vi "Coerce Scale Range to Content.vi"(8 "error in (no error)":errorcluster, 11 "Base Graph in":refnum<class "Base Graph.lvclass">) -> (0 "error out":errorcluster, 3 "Base Graph out":refnum<class "Base Graph.lvclass">)   [LabVIEW 2023, in "Base Graph.lvclass"]
uses:
  Base Graph.lvclass
  Base Graph.lvclass/Base Graph.ctl
panel:
  # "AFTER DEZOOMING THE INTENSITY GRAPH IS 1PIXEL TO BIG"
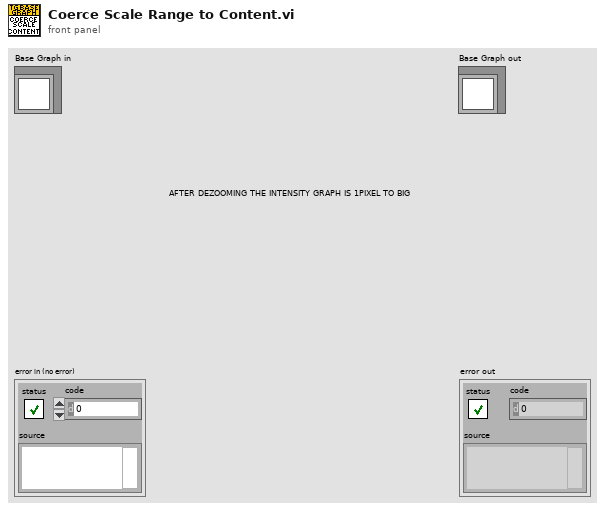
[diagram p1: front panel]
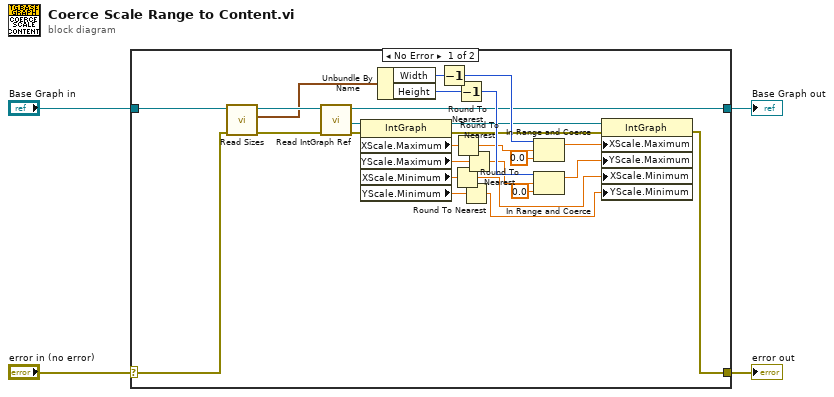
[diagram p0: block diagram]
diagram:
  n1 = case shown="No Error" "error in (no error)" {
    selector: "error in (no error)" -> [w26 w33]
    tunnel: [w13 w33] -> w3
    tunnel: [w14 w32] -> w1
    tunnel: "Base Graph in" -> [w31 w32]
    frame No Error {
      n2 = call "Read Sizes.vi"("error in (no error)"=w26, "TG Base Graph in"=w31) -> ("error out"=w27:errorcluster, "Sizes"=w28:cluster{"Height":u32, "Width":u32}, "TG Base Graph out"=w30:refnum<class "Base Graph.lvclass">)  [unwired: 7 in]
      n3 = call "Read IntGraph Ref.vi"("error in (no error)"=w27, "TG Base Graph in"=w30) -> ("error out"=w25:errorcluster, "IntGraph Ref"=w29:refnum<vi>, "TG Base Graph out"=w14:refnum<class "Base Graph.lvclass">)  [unwired: 7 in]
      n4 = property class="IntGraph"(reference=w29, error in=w25) -> (reference out=w16:refnum<vi>, error out=w15:errorcluster, "XScale.Maximum"=w24:dbl, "YScale.Maximum"=w20:dbl, "XScale.Minimum"=w10:dbl, "YScale.Minimum"=w9:dbl)
      n5 = Unbundle By Name(w28) -> ("Width"=w23:u32, "Height"=w19:u32)
      n6 = Decrement(x=w23) -> (x-1=w22:u32)
      n7 = Round To Nearest(number=w10) -> (nearest integer value=w6:dbl)
      n8 = Round To Nearest(number=w24) -> (nearest integer value=w8:dbl)
      n9 = Decrement(x=w19) -> (x-1=w18:u32)
      n10 = Round To Nearest(number=w9) -> (nearest integer value=w5:dbl)
      n11 = Round To Nearest(number=w20) -> (nearest integer value=w7:dbl)
      n12 = In Range and Coerce(upper limit=w22, x=w8, lower limit=0.0) -> (coerced(x)=w12:dbl)  [unwired: 1 out]
      n13 = In Range and Coerce(upper limit=w18, x=w7, lower limit=0.0) -> (coerced(x)=w11:dbl)  [unwired: 1 out]
      n14 = property class="IntGraph"(reference=w16, error in=w15, "XScale.Maximum"=w12, "YScale.Maximum"=w11, "XScale.Minimum"=w6, "YScale.Minimum"=w5) -> (error out=w13:errorcluster)  [unwired: 1 out]
    }
    frame Error {
    }
  }
  "error out" <- w3
  "Base Graph out" <- w1
